vi "y cut IV.vi"(6 "Contact Resistance":dbl, 8 "x offset":dbl, 9 "x pos":dbl, 10 "scale":dbl, 11 "Data":dbl[][](array[numeric])) -> (1 "Y":dbl[](array[numeric]), 2 "X":dbl[](array[numeric]), 3 "IV":cluster{"Data":dbl[], dbl[]})   [LabVIEW 2024]
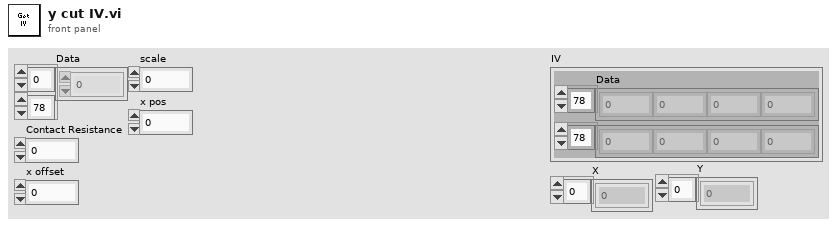
[diagram p1: front panel]
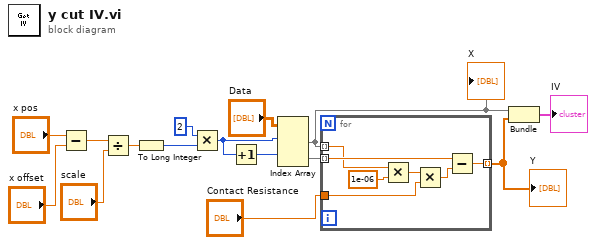
[diagram p0: block diagram]
diagram:
  n1 = Subtract(x="x pos", y="x offset") -> (x-y=w15:dbl)
  n2 = Divide(x=w15, y="scale") -> (x/y=w14:dbl)
  n3 = To Long Integer(number=w14) -> (32bit integer=w10:i32)
  n4 = Multiply(x=2, y=w10) -> (x*y=w12:i32)
  n5 = Increment(x=w12) -> (x+1=w11:i32)
  n6 = Index Array(array="Data", index (row) #1=w12, index (row) #2=w11) -> (element #1=w7:dbl[], element #2=w9:dbl[])  [unwired: 2 in]
  "X" <- w7
  n7 = for {
    tunnel: w9 -> [w22] mode=indexing
    tunnel: w7 -> [w21] mode=indexing
    tunnel: [w19] -> w8 mode=indexing
    tunnel: "Contact Resistance" -> [w16]
    n8 = Multiply(x=w21, y=1e-06 ("x")) -> (x*y=w18:dbl)
    n9 = Multiply(x=w18, y=w16) -> (x*y=w20:dbl)
    n10 = Subtract(x=w22, y=w20) -> (x-y=w19:dbl)
  }
  "Y" <- w8
  n11 = Bundle("Data"=w7, w8) -> (→"IV":cluster{"Data":dbl[], dbl[]})  [unwired: 1 in]
